vi "Evaluate_Force.vi"() -> ()   [LabVIEW 2015]
uses:
  <instrlib>/Dynamixel Motor/Public/Motor Operation/Low Level/Baud Setting.ctl
  <instrlib>/Dynamixel Motor/Dynamixel Motor.lvlib
panel:
  in  "Position Data Filename":path=path "C:/Users/utente/Documents/UB/TESI/Force_Evaluation_ultimo_pollice44_no_peso/test_position_pollice44_no_peso.xlsx"
  in  "Current Data Filename":path=path "C:/Users/utente/Documents/UB/TESI/Force_Evaluation_ultimo_pollice44_no_peso/test_current_pollice44_no_peso.xlsx"
  in  "Stop Button":bool
  in  "input cluster 2":cluster{"Load":dbl}
  in  "input cluster":cluster{"Load":dbl}
  out "Current load":dbl[](array[numeric])
  out "Position":dbl[](array[numeric])
  out "error out":errorcluster
  in  "VISA resource name":refnum<visa-resource-name>="COM9"
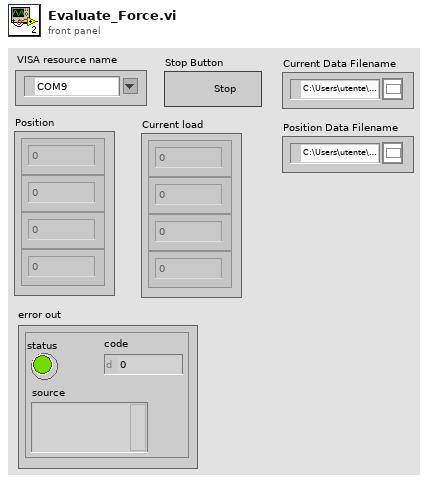
[diagram p1: front panel]
types:
  T1 = typedef "Dynamixel Motor.lvlib/Baud Setting.ctl" = u8
  T2 = typedef "Real Matrix NI_Silver.ctl" = dbl[][]
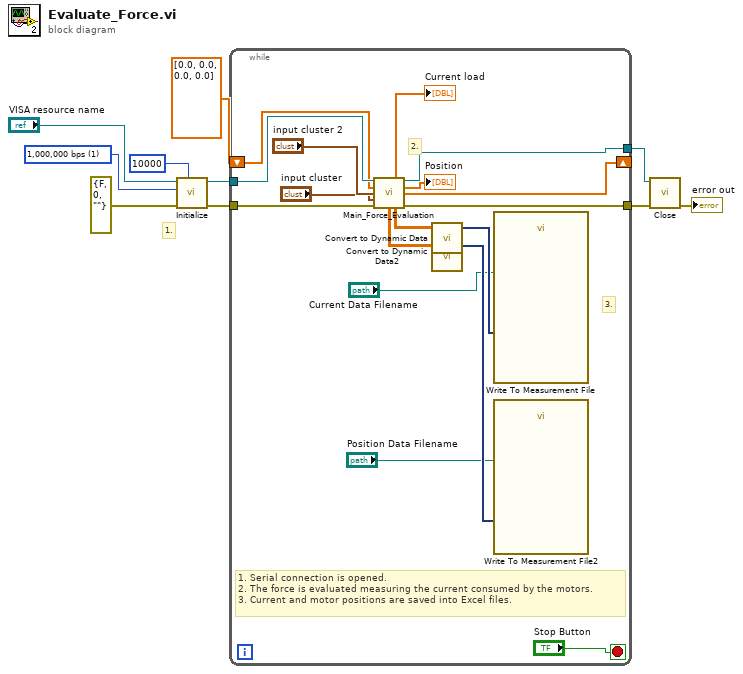
[diagram p0: block diagram]
diagram:
  w10 = T1 1 items=["1,000,000 bps"=1, "500,000 bps"=3, "400,000 bps"=4, "250,000 bps"=7, "200,000 bps"=9, "115200 bps"=16, "57600 bps"=34, "19200 bps"=103, "9600 bps"=207] ("Baud rate (57600 bps)")
  # "1."
  n1 = call <instrlib>:"Initialize.vi"("Timeout (30 msec)"=u32 10000, "error in (no error)"=errorcluster {"status"=FALSE, "code"=0, "source"=""}, "Baud rate (57600 bps)"=w10, "VISA resource name"="VISA resource name") -> ("error out"=w4:errorcluster, "VISA resource name out"=w5:refnum<visa-resource-name>)  [unwired: 6 in]
  n2 = while {
    tunnel: w5 -> [w27]
    tunnel: w4 -> [w26]
    shift-right: [w17] -> _
    shift-left: dbl[] [0.0, 0.0, 0.0, 0.0] -> [w25]
    tunnel: [w24] -> w2
    tunnel: [w23] -> w1
    stop <- "Stop Button" stop-if-true
    # "3."
    # "2."
    # "1. Serial connection is opened.\n2. The force is evaluated measuring the current consumed by the motors.\n3. Current and motor positions are saved into Excel files."
    n3 = call "Main_Force_Evaluation.vi"("VISA Refnum in"=w27, "Positions to reach"=w25, "Store cluster position"="input cluster 2", "Store cluster current"="input cluster", "error in (no error)"=w26) -> ("Current (mA)"=→"Current load":dbl[], "VISA Refnum out"=w24:refnum<visa-resource-name>, "Actual positions"=→"Position":dbl[], "New positions to reach"=w17:dbl[], "Positions to Excel"=w13:T2, "Currents to Excel"=w14:T2, "error out"=w23:errorcluster)  [unwired: 4 in]
    n4 = call "Convert to Dynamic Data"("2D Array"=w14) -> ("Dynamic Data Type"=w22:dynamicdata)  [unwired: 3 in]
    n5 = call "Convert to Dynamic Data2"("2D Array"=w13) -> ("Dynamic Data Type"=w21:dynamicdata)  [unwired: 3 in]
    n6 = call "Write To Measurement File"("Signals"=w22, "Filename"="Current Data Filename") -> ()  [unwired: 15 in, 3 out]
    n7 = call "Write To Measurement File2"("Signals"=w21, "Filename"="Position Data Filename") -> ()  [unwired: 15 in, 3 out]
  }
  n8 = call <instrlib>:"Close.vi"("error in (no error)"=w1, "VISA resource name"=w2) -> ("error out"=→"error out":errorcluster)  [unwired: 9 in]
